vi "Osciloscope.vi"(3 "Waveform Graph":waveform(dbl)(graph)) -> ()   [LabVIEW 2024]
uses:
  <vilib>/Utility/miscctls.llb/LVRangeTypeDef.ctl
panel:
  in  "Time/div":dbl(knob) min=0.0 max=0.1 step=0.001 scale=0.0001..0.1
  in  "DC":dbl(knob) scale=0.0..10.0
  in  "V/div":dbl(knob)=0.1 min=0.1 max=10.0 step=0.01 scale=0.1..10.0
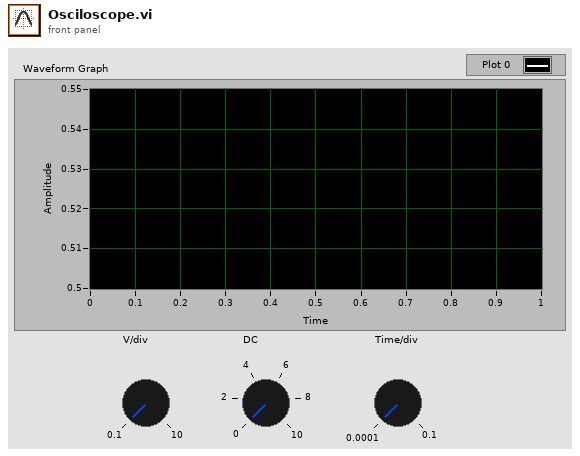
[diagram p1: front panel]
types:
  T1 = typedef "LVRangeTypeDef.ctl" = cluster{"Minimum":dbl, "Maximum":dbl, "Increment":dbl, "Minor Increment":dbl, "Start":dbl}
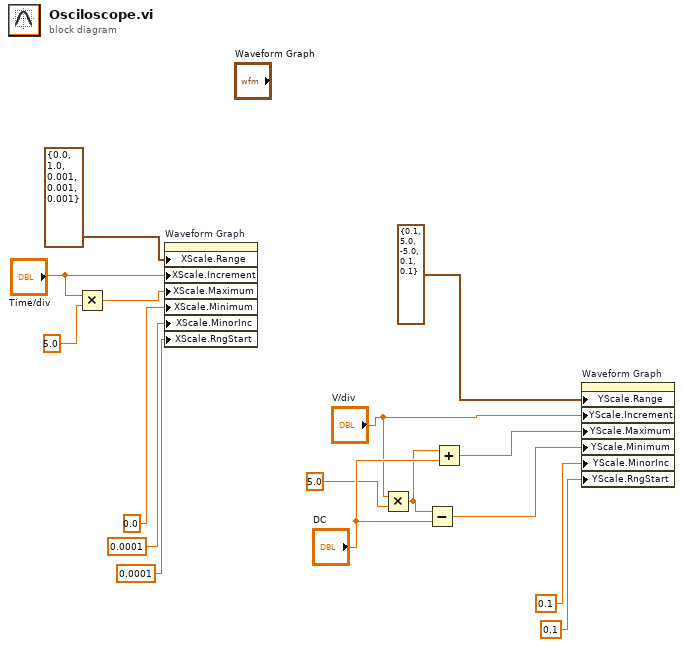
[diagram p0: block diagram]
diagram:
  n1 = Multiply(x="Time/div", y=5.0) -> (x*y=w8:dbl)
  n2 = property on="Waveform Graph" class="WFGraph (strict)"("XScale.Range"=T1 {"Minimum"=0.0, "Maximum"=1.0, "Increment"=0.001, "Minor Increment"=0.001, "Start"=0.001} ("X Scale.Range"), "XScale.Increment"="Time/div", "XScale.Maximum"=w8, "XScale.Minimum"=0.0 ("X Scale.Range:Minimum"), "XScale.MinorInc"=0.0001 ("X Scale.Range:Minor Increment"), "XScale.RngStart"=0.0001 ("X Scale.Range:Start")) -> ()  [unwired: 2 in, 2 out]
  n3 = Multiply(x="V/div", y=5.0 ("Y Scale.Range:Increment")) -> (x*y=w3:dbl)
  n4 = Subtract(x=w3, y="DC") -> (x-y=w9:dbl)
  n5 = Add(x=w3, y="DC") -> (x+y=w5:dbl)
  n6 = property on="Waveform Graph" class="WFGraph (strict)"("YScale.Range"=T1 {"Minimum"=0.1, "Maximum"=5.0, "Increment"=-5.0, "Minor Increment"=0.1, "Start"=0.1} ("Y Scale.Range"), "YScale.Increment"="V/div", "YScale.Maximum"=w5, "YScale.Minimum"=w9, "YScale.MinorInc"=0.1 ("Y Scale.Range:Minor Increment"), "YScale.RngStart"=0.1 ("Y Scale.Range:Start")) -> ()  [unwired: 2 in, 2 out]
